vi "IO_Tank_Control.vi"() -> ()   [LabVIEW 2024]
doc: "This example performs writes and reads on a serial port, as directed by the user. You can press the Write and Read buttons, and change the Read Count, while the example is running.\n\nThe parameters set for the serial port must match the parameters of the connected instrument or device. In this example, the Read Count parameter specifies the number of bytes that the serial port reads. If there were more bytes at the port than the specified number, those bytes would not be read. If there were less bytes at the port than the specified number, you would receive a timeout error.\n\nThis example expands upon the flow control options for XON and XOFF, allowing the user to choose those control characters. Also, the user can enable or disable a termination character. Some devices require a termination character in order to identify the end of command strings. Some devices send a termination character to signify the end of data to be read. This example shows how you can end the Read operation once a termination character is detected in the buffer and/or append a termination character at the end of the Write data."
uses:
  LabVIEW_InstrDriver_forLK-G3000_ver1_0_1_0/32bit/Keyence LK-G3000/Public/clusters/LKIF_FLOATVALUE.ctl
  LabVIEW_InstrDriver_forLK-G3000_ver1_0_1_0/32bit/Keyence LK-G3000/Public/enums/LKIF_FLOATRESULT.ctl
  <vilib>/Instr/_visa.llb/VISA Configure Serial Port (Instr).vi
  LabVIEW_InstrDriver_forLK-G3000_ver1_0_1_0/32bit/Keyence LK-G3000/Keyence LK-G3000.lvlib
panel:
  out "CalcData2":T1 {"LKIF_FLOATRESULT" items=["VALID", "RANGEOVER_P", "RANGEOVER_N", "WAITING"]}
  out "CalcData1":T1 {"LKIF_FLOATRESULT" items=["VALID", "RANGEOVER_P", "RANGEOVER_N", "WAITING"]}
  out "Trend Graph":cluster{"Value":sgl, "Value":sgl}(graph)
  out "Read Buffer":string[](array[string])
  in  "STOP":bool
  in  "DRAIN":bool
  in  "FILL":bool
  in  "Stop Button":bool
  in  "State":enum16{"INIT", "IDLE", "STOP", "FILL", "DRAIN"}(ring)
  out "Numeric":i32=2
  in  "2108 CDC Virtual COM":refnum<visa-resource-name>="COM3"
  # "Analog In\n\nencode 0\nslist 0 0\nslist 1 1\nsrate 6000\nps 2\ndec 1\ndeca 3\nnop"
  # "encode 0\nslist 0 0\nslist 1 1\nsrate 6000\nps 2\ndec 1\ndeca 3\nnop"
  # "encode 0 Enables the binary output mode (DEFAULT"
  # "info 0    Returns \"info 0 DATAQ\"\ninfo 1    Returns device model number (e.g.\"info 1 2008\")\ninfo 2    Returns firmware revision, 2 hex bytes (e.g. 6516 = 10110 for firmware revision 1.01)\ninfo 3    to info 4 Proprietary internal use for initial system verification\ninfo 5    <arg0>\n            Sets device description string arg0 (31 characters followed by null). Issued without <arg0> returns the \n            previously defined device description string. arg0 may be contained within quotation marks to included spaces \n            in device description. Model DI-2008 does not support info 5.\ninfo 6    Returns the instrument's serial number (left-most 8 digits only)\ninfo 7    to info 8 Proprietary internal use for initial system verification\ninfo 9    Returns the sample rate dividend value based upon current settings (see the srate command for details"
  # "0x60 = 96   FILL\n0x40 = 64  OFF\n0x20 = 32  DRAIN\n0x00 = 00  OFF"
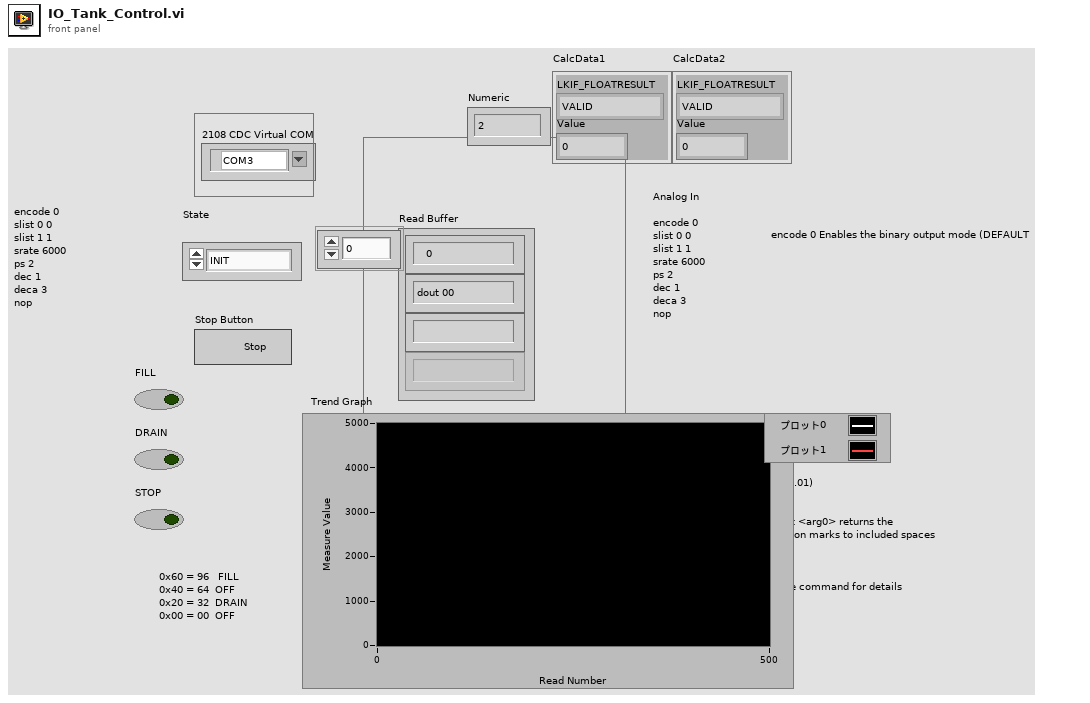
[diagram p1: front panel]
types:
  T1 = typedef "Keyence LK-G3000.lvlib/LKIF_FLOATVALUE.ctl" = cluster{"LKIF_FLOATRESULT":T2, "Value":sgl}
  T2 = typedef "Keyence LK-G3000.lvlib/LKIF_FLOATRESULT.ctl" = i32
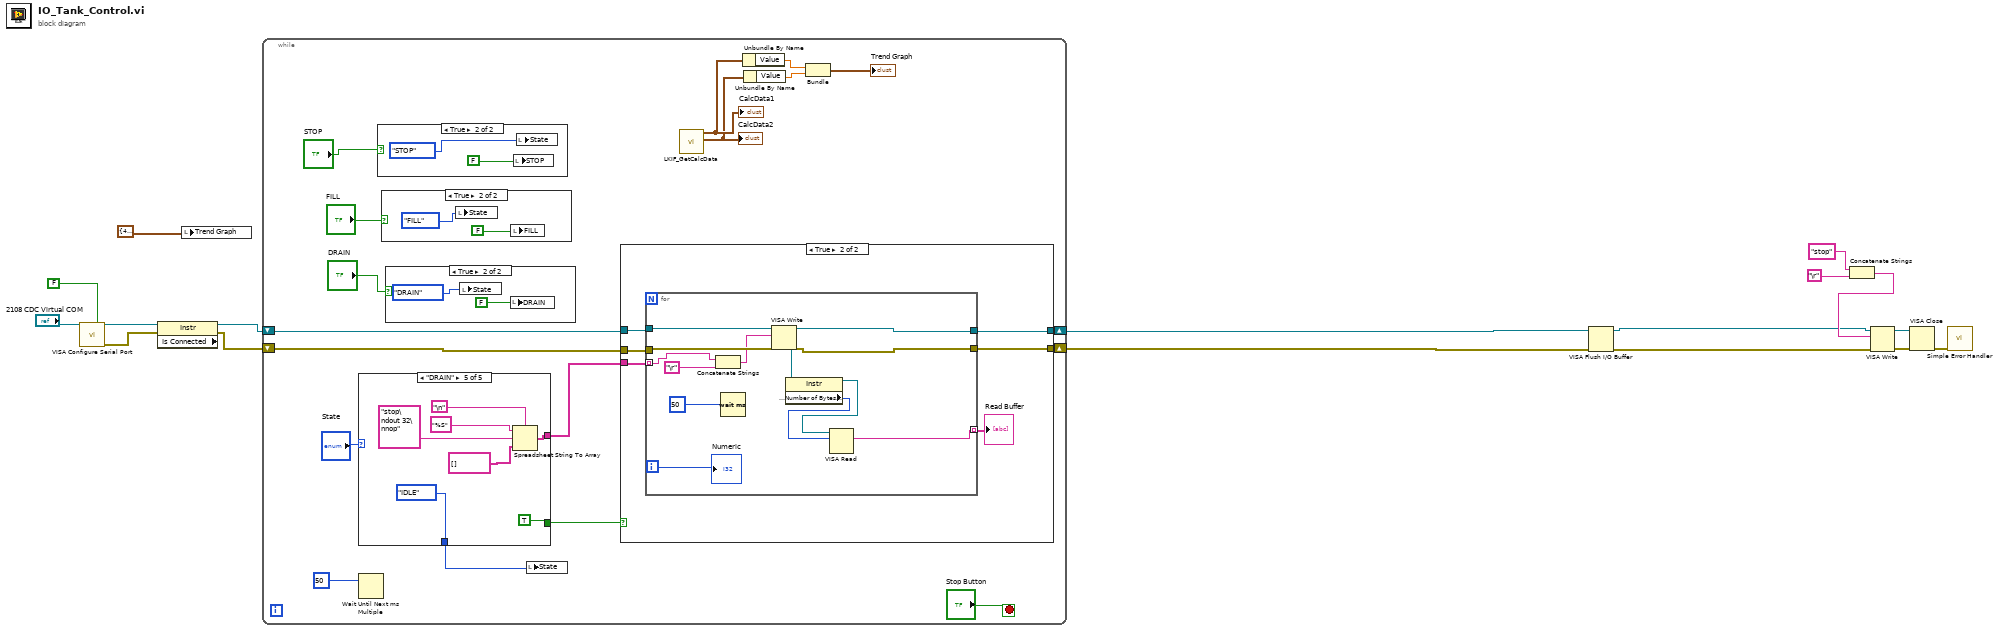
[diagram p0: block diagram]
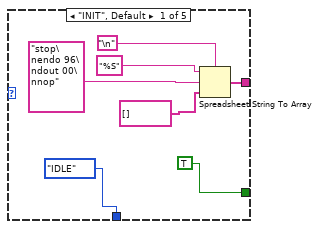
[diagram p6: hidden frame]
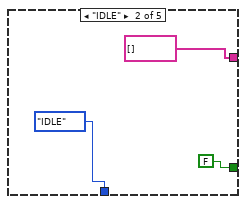
[diagram p7: hidden frame]
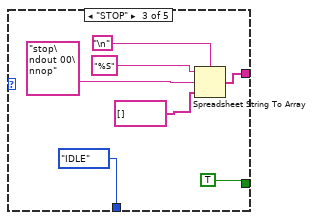
[diagram p8: hidden frame]
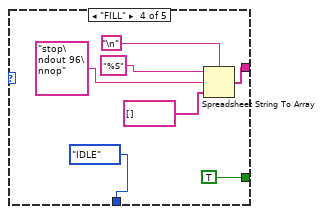
[diagram p9: hidden frame]
diagram:
  n1 = call-poly "VISA Configure Serial Port"("VISA resource name"="2108 CDC Virtual COM", "Enable Termination\nChar (T)"=FALSE) -> ("VISA resource name out"=w15:refnum<visa-resource-name>, "error out"=w17:errorcluster)  [unwired: 8 in, 4 out]
  n2 = property class="Instr" props=["Is Connected"](reference=w15, error in=w17) -> (reference out=w5:refnum<visa-resource-name>, error out=w4:errorcluster)  [unwired: 1 out]
  n3 = local write "Trend Graph"(cluster{"Value":sgl, "Value":sgl} {"Value"=4.6782, "Value"=4678.4} ("Trend Graph")) -> ()
  n4 = while {
    shift-right: [w35] -> w7
    shift-left: w5 -> [w33]
    shift-right: [w34] -> w6
    shift-left: w4 -> [w32]
    stop <- "Stop Button" stop-if-true
    n5 = case shown="\"DRAIN\"" "State" {
      tunnel: [w65 string[] [] w74 w81 w87] -> w23
      tunnel: [TRUE FALSE TRUE TRUE TRUE] -> w30
      tunnel: [enum16{"INIT", "IDLE", "STOP", "FILL", "DRAIN"}."IDLE" ("State") enum16{"INIT", "IDLE", "STOP", "FILL", "DRAIN"}."IDLE" ("State") enum16{"INIT", "IDLE", "STOP", "FILL", "DRAIN"}."IDLE" ("State") enum16{"INIT", "IDLE", "STOP", "FILL", "DRAIN"}."IDLE" ("State") enum16{"INIT", "IDLE", "STOP", "FILL", "DRAIN"}."IDLE" ("State")] -> w29
      frame "INIT", Default {
        n6 = Spreadsheet String To Array(delimiter (Tab)="\n", format string="%S", spreadsheet string="stop\nendo 96\ndout 00\nnop" ("Command List"), array type (2D Dbl)=string[] []) -> (array=w65:string[])
      }
      frame "IDLE" {
      }
      frame "STOP" {
        n7 = Spreadsheet String To Array(delimiter (Tab)="\n", format string="%S", spreadsheet string="stop\ndout 00\nnop" ("Command List"), array type (2D Dbl)=string[] []) -> (array=w74:string[])
      }
      frame "FILL" {
        n8 = Spreadsheet String To Array(delimiter (Tab)="\n", format string="%S", spreadsheet string="stop\ndout 96\nnop" ("Command List"), array type (2D Dbl)=string[] []) -> (array=w81:string[])
      }
      frame "DRAIN" {
        n9 = Spreadsheet String To Array(delimiter (Tab)="\n", format string="%S", spreadsheet string="stop\ndout 32\nnop" ("Command List"), array type (2D Dbl)=string[] []) -> (array=w87:string[])
      }
    }
    n10 = Wait Until Next ms Multiple(millisecond multiple=50) -> ()  [unwired: 1 out]
    n11 = case shown="True" "STOP" {
      frame False {
      }
      frame True {
        n12 = local write "STOP"(FALSE ("FILL")) -> ()
        n13 = local write "State"(enum16{"INIT", "IDLE", "STOP", "FILL", "DRAIN"}."STOP" ("State")) -> ()
      }
    }
    n14 = case shown="True" "FILL" {
      frame False {
      }
      frame True {
        n15 = local write "State"(enum16{"INIT", "IDLE", "STOP", "FILL", "DRAIN"}."FILL" ("State")) -> ()
        n16 = local write "FILL"(FALSE ("FILL")) -> ()
      }
    }
    n17 = case shown="True" "DRAIN" {
      frame False {
      }
      frame True {
        n18 = local write "State"(enum16{"INIT", "IDLE", "STOP", "FILL", "DRAIN"}."DRAIN" ("State")) -> ()
        n19 = local write "DRAIN"(FALSE ("FILL")) -> ()
      }
    }
    n20 = local write "State"(w29) -> ()
    n21 = case shown="True" w30 {
      tunnel: [w43 w49] -> w35
      tunnel: [w42 w48] -> w34
      tunnel: w33 -> [w43 w47]
      tunnel: w32 -> [w42 w46]
      tunnel: w23 -> [_ w45]
      frame False {
      }
      frame True {
        n22 = for {
          tunnel: w45 -> [w59] mode=indexing
          tunnel: w47 -> [w61]
          tunnel: w46 -> [w60]
          tunnel: [w57] -> w49
          tunnel: [w58] -> w48
          tunnel: [w50] -> w44 mode=indexing
          i -> [w56]
          n23 = Concatenate Strings(w59, "\r") -> (w53:string)
          n24 = Wait (ms)(milliseconds to wait=u32 50) -> ()  [unwired: 1 out]
          n25 = VISA Write(VISA resource name=w61, write buffer=w53, error in (no error)=w60) -> (VISA resource name out=w57:refnum<visa-resource-name>, error out=w58:errorcluster)  [unwired: 1 out]
          n26 = property class="Instr"(reference=w57) -> (reference out=w52:refnum<visa-resource-name>, "Serial Settings:Number of Bytes at Serial Port"=w51:u32)  [unwired: 1 in, 1 out]
          n27 = VISA Read(VISA resource name=w52, byte count=w51) -> (read buffer=w50:string)  [unwired: 1 in, 3 out]
          "Numeric" <- w56
        }
        "Read Buffer" <- w44
      }
    }
    n28 = call "LKIF_GetCalcData.vi"() -> ("CalcData2"=w21:T1, "CalcData1"=w22:T1)  [unwired: 9 in, 1 out]
    "CalcData1" <- w22
    "CalcData2" <- w21
    n29 = Unbundle By Name(w22) -> ("Value"=w20:sgl)
    n30 = Unbundle By Name(w21) -> ("Value"=w19:sgl)
    n31 = Bundle("Value"=w20, "Value"=w19) -> (→"Trend Graph":cluster{"Value":sgl, "Value":sgl})  [unwired: 1 in]
  }
  n32 = VISA Flush I/O Buffer(VISA resource name=w7, error in (no error)=w6) -> (VISA resource name out=w3:refnum<visa-resource-name>, error out=w2:errorcluster)  [unwired: 1 in]
  n33 = Concatenate Strings("stop", "\r") -> (w9:string)
  n34 = VISA Write(VISA resource name=w3, write buffer=w9, error in (no error)=w2) -> (VISA resource name out=w13:refnum<visa-resource-name>, error out=w12:errorcluster)  [unwired: 1 out]
  n35 = VISA Close(VISA resource name=w13, error in (no error)=w12) -> (error out=w16:errorcluster)
  n36 = call <vilib>:"Simple Error Handler.vi"("error in (no error)"=w16) -> ()  [unwired: 1 in, 8 out]
